vi "获取绑定信息.vi"() -> ()   [LabVIEW 2013, in "数据库操作.lvclass"]
uses:
  <vilib>/addons/database/Connection.llb/Conn ObjectReference.ctl
  <vilib>/addons/database/NI_Database_API.lvlib
panel:
  in  "用户名":string
  in  "数据库连接引用":T1
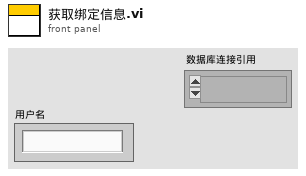
[diagram p1: front panel]
types:
  T1 = typedef "NI_Database_API.lvlib/Conn ObjectReference.ctl" = refnum<k1>
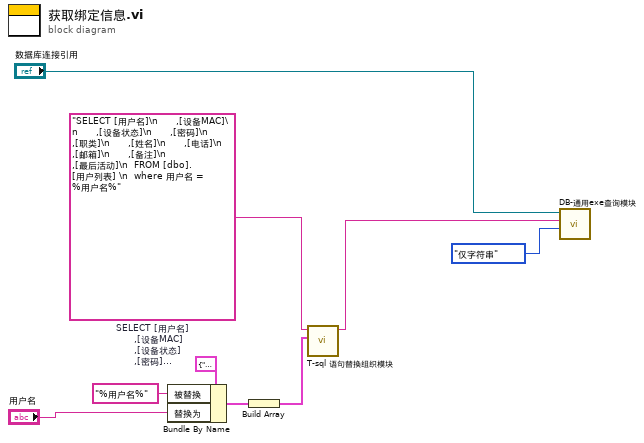
[diagram p0: block diagram]
diagram:
  w7 = "SELECT [用户名]\n      ,[设备MAC]\n      ,[设备状态]\n      ,[密码]\n      ,[职类]\n      ,[姓名]\n      ,[电话]\n      ,[邮箱]\n      ,[备注]\n      ,[最后活动]\n  FROM [dbo].[用户列表] \n  where 用户名 = %用户名%"  # SELECT [用户名]       ,[设备MAC]       ,[设备状态]       ,[密码]       ,[职类]       ,[姓名]       ,[电话]       ,[邮箱]       ,[备注]       ,[最后活动]   FROM [dbo].[用户列表]    where 用户名 = %用户名%
  n1 = Bundle By Name(cluster=cluster{"被替换":string, "替换为":string} {"被替换"="", "替换为"=""} ("替换单元"), "被替换"="%用户名%", "替换为"="用户名") -> (w3:cluster{"被替换":string, "替换为":string})
  n2 = Build Array(w3) -> (w2:cluster{"被替换":string, "替换为":string}[])
  n3 = call "T-sql 语句替换组织模块.vi"("替换项"=w2, "T-sql 模板"=w7) -> ("T-sql"=w1:string)  [unwired: 8 in, 1 out]
  n4 = call "DB-通用exe查询模块.vi"("解析模式"=enum16{"仅数值", "仅字符串", "数值与字符串"}."仅字符串", "SQL query"=w1, "数据库连接引用"="数据库连接引用") -> ()  [unwired: 5 in, 4 out]
